vi "Configure System (Information).vi"(7 "Scanner Interface (F:Disable)":bool, 8 "error in (no error)":errorcluster, 9 "Handler Interface (F:Disable)":bool, 10 "Current Bias Interface (F:Disable)":bool, 11 "VISA resource name":refnum<visa-resource-name>) -> (0 "error out":errorcluster, 3 "VISA resource name out":refnum<visa-resource-name>)   [LabVIEW 2016, in "Agilent E4980.lvlib"]
doc: "Enables or disables the bias current interface, the handler interface, and the scanner interfacae."
uses:
  <instrlib>/Agilent E4980/Agilent E4980.lvlib
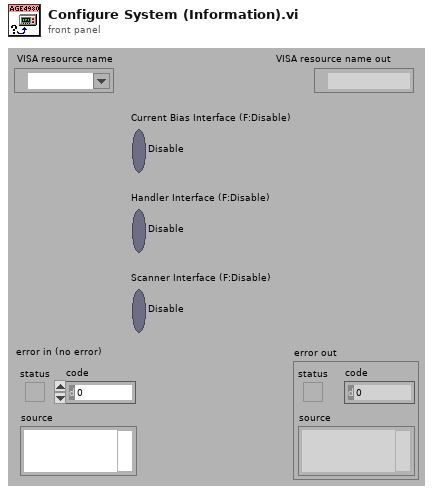
[diagram p1: front panel]
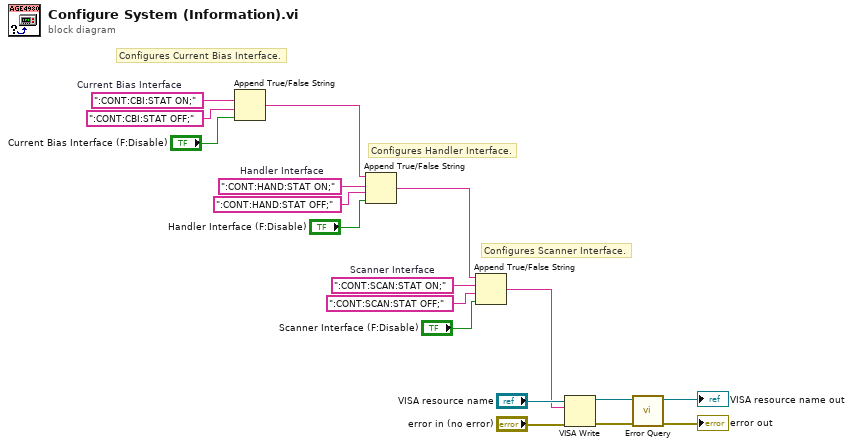
[diagram p0: block diagram]
diagram:
  w12 = ":CONT:SCAN:STAT ON;"  # Scanner Interface
  w15 = ":CONT:HAND:STAT ON;"  # Handler Interface
  w18 = ":CONT:CBI:STAT ON;"  # Current Bias Interface
  # "Configures Scanner Interface."
  # "Configures Handler Interface."
  # "Configures Current Bias Interface."
  n1 = Append True/False String(1:"Current Bias Interface (F:Disable)", 2:":CONT:CBI:STAT OFF;" ("false string"), 3:w18) -> (0:w2:string)  [unwired: 1 in]
  n2 = Append True/False String(1:"Handler Interface (F:Disable)", 2:":CONT:HAND:STAT OFF;" ("false string"), 3:w15, 4:w2) -> (0:w3:string)
  n3 = Append True/False String(1:"Scanner Interface (F:Disable)", 2:":CONT:SCAN:STAT OFF;" ("false string"), 3:w12, 4:w3) -> (0:w1:string)
  n4 = VISA Write(VISA resource name="VISA resource name", write buffer=w1, error in (no error)="error in (no error)") -> (VISA resource name out=w7:refnum<visa-resource-name>, error out=w6:errorcluster)  [unwired: 1 out]
  n5 = call <instrlib>:"Error Query.vi"("error in (no error)"=w6, "VISA resource name"=w7) -> ("error out"=→"error out":errorcluster, "VISA resource name out"=→"VISA resource name out":refnum<visa-resource-name>)  [unwired: 6 in, 2 out]
